vi "Keithley1a_230X_Setting.vi"(11 "YTESTER测试数据":T1) -> (3 "YTESTER结论":T2)   [LabVIEW 2017]
uses:
  YtCommon.lvlibp/yt`Step StepBaseInput.ctl
  YtCommon.lvlibp/yt`Step StepResult.ctl
  YtCommon.lvlibp/yt`Step TestData.ctl
  YtCommon.lvlibp/yt`Step System Queue.ctl
  YtCommon.lvlibp
panel:
  in  "YTESTER开放参数":T4={"YTESTER_BaseInput"={"isTest"=FALSE, "isSkip"=FALSE, "StepName"="Keithley230X设置", "OnPass"=enum."Next", "OnFail"=enum."Next", "ReTestNumber"=0.0}, "VISA resource"="", "设置选择"=enum."设置 CH1 电压&限流", "设置电压（V）"=5.0, "设置限流（mA）"=50.0}
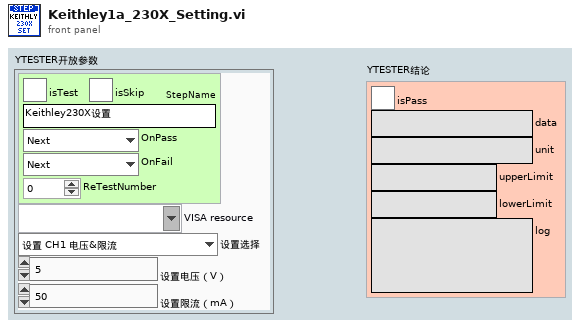
[diagram p1: front panel]
types:
  T1 = typedef "YtCommon.lvlibp/yt`Step TestData.ctl" = cluster{"Socket(From1)":i32, "SN":refnum<notifier>, "StopFlagRef":refnum<notifier>, "YT System Queue":refnum<queue>}
  T2 = typedef "YtCommon.lvlibp/yt`Step StepResult.ctl" = cluster{"isPass":bool, "data":string, "unit":string, "upperLimit":string, "lowerLimit":string, "log":string}
  T3 = typedef "YtCommon.lvlibp/yt`Step StepBaseInput.ctl" = cluster{"isTest":bool, "isSkip":bool, "StepName":string, "OnPass":enum16{"Next", "ToOVER", "Terminate"}, "OnFail":enum16{"Next", "ToOVER", "Terminate"}, "ReTestNumber":dbl}
  T4 = cluster{"YTESTER_BaseInput":T3, "VISA resource":refnum<visa-resource-name>, "设置选择":enum16{"设置 CH1 电压&限流", "设置 CH2 电压&限流", "打开 CH1", "打开 CH2", "关闭 CH1", "关闭 CH2", "打开 全部", "关闭 全部", "打开 屏显", "关闭 屏显", "查询设备（IDN？）"}, "设置电压（V）":dbl, "设置限流（mA）":dbl}
  T5 = enum16{"设置 CH1 电压&限流", "设置 CH2 电压&限流", "打开 CH1", "打开 CH2", "关闭 CH1", "关闭 CH2", "打开 全部", "关闭 全部", "打开 屏显", "关闭 屏显", "查询设备（IDN？）"}
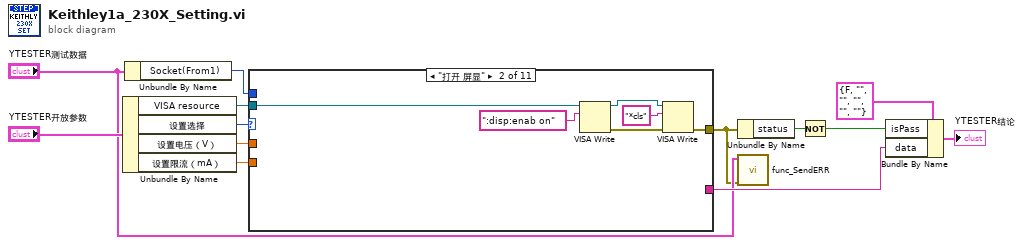
[diagram p0: block diagram]
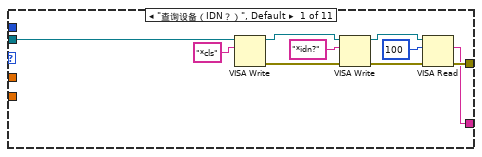
[diagram p2: hidden frame]
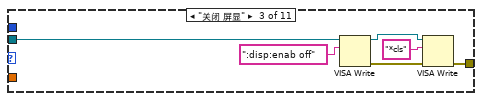
[diagram p3: hidden frame]
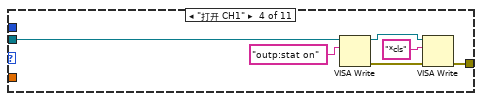
[diagram p4: hidden frame]
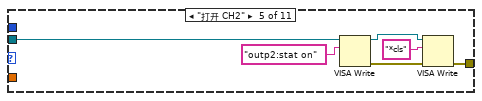
[diagram p5: hidden frame]
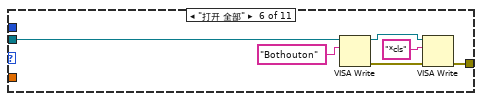
[diagram p6: hidden frame]
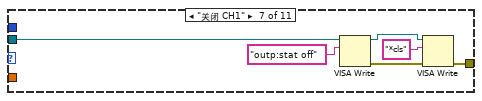
[diagram p7: hidden frame]
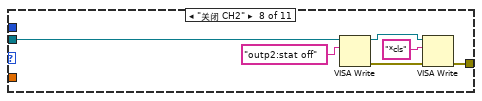
[diagram p8: hidden frame]
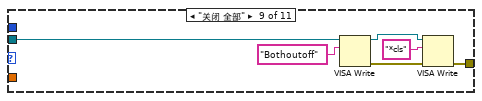
[diagram p9: hidden frame]
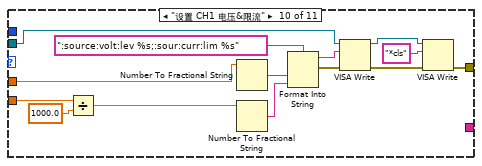
[diagram p10: hidden frame]
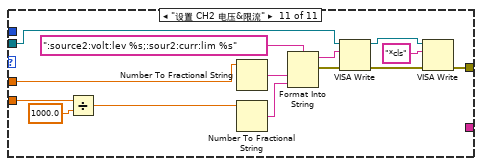
[diagram p11: hidden frame]
diagram:
  n1 = Unbundle By Name("YTESTER开放参数") -> ("VISA resource"=w9:refnum<visa-resource-name>, "设置选择"=w10:T5, "设置电压（V）"=w8:dbl, "设置限流（mA）"=w7:dbl)
  n2 = Unbundle By Name("YTESTER测试数据") -> ("Socket(From1)"=w4:i32)
  n3 = case shown="\"打开 屏显\"" w10 {
    tunnel: w9 -> [w16 w24 w31 w36 w43 w50 w55 w61 w67 w73 w89]
    tunnel: [w15 w25 w30 w37 w42 w48 w54 w60 w66 w72 w86] -> w3
    tunnel: w8 -> [_ _ _ _ _ _ _ _ _ w82 w88]
    tunnel: w7 -> [_ _ _ _ _ _ _ _ _ w79 w87]
    tunnel: [w14 _ _ _ _ _ _ _ _ _ _] -> w6
    tunnel: w4 -> [_ _ _ _ _ _ _ _ _ _ _]
    frame "查询设备（IDN？）", Default {
      n4 = VISA Write(VISA resource name=w16, write buffer="*cls") -> (VISA resource name out=w22:refnum<visa-resource-name>, error out=w18:errorcluster)  [unwired: 1 in, 1 out]
      n5 = VISA Write(VISA resource name=w22, write buffer="*idn?", error in (no error)=w18) -> (VISA resource name out=w20:refnum<visa-resource-name>, error out=w19:errorcluster)  [unwired: 1 out]
      n6 = VISA Read(VISA resource name=w20, byte count=u32 100, error in (no error)=w19) -> (read buffer=w14:string, error out=w15:errorcluster)  [unwired: 2 out]
    }
    frame "打开 屏显" {
      n7 = VISA Write(VISA resource name=w24, write buffer=":disp:enab on") -> (VISA resource name out=w28:refnum<visa-resource-name>, error out=w27:errorcluster)  [unwired: 1 in, 1 out]
      n8 = VISA Write(VISA resource name=w28, write buffer="*cls", error in (no error)=w27) -> (error out=w25:errorcluster)  [unwired: 2 out]
    }
    frame "关闭 屏显" {
      n9 = VISA Write(VISA resource name=w31, write buffer=":disp:enab off") -> (VISA resource name out=w34:refnum<visa-resource-name>, error out=w33:errorcluster)  [unwired: 1 in, 1 out]
      n10 = VISA Write(VISA resource name=w34, write buffer="*cls", error in (no error)=w33) -> (error out=w30:errorcluster)  [unwired: 2 out]
    }
    frame "打开 CH1" {
      n11 = VISA Write(VISA resource name=w36, write buffer="outp:stat on") -> (VISA resource name out=w40:refnum<visa-resource-name>, error out=w38:errorcluster)  [unwired: 1 in, 1 out]
      n12 = VISA Write(VISA resource name=w40, write buffer="*cls", error in (no error)=w38) -> (error out=w37:errorcluster)  [unwired: 2 out]
    }
    frame "打开 CH2" {
      n13 = VISA Write(VISA resource name=w43, write buffer="outp2:stat on") -> (VISA resource name out=w46:refnum<visa-resource-name>, error out=w44:errorcluster)  [unwired: 1 in, 1 out]
      n14 = VISA Write(VISA resource name=w46, write buffer="*cls", error in (no error)=w44) -> (error out=w42:errorcluster)  [unwired: 2 out]
    }
    frame "打开 全部" {
      n15 = VISA Write(VISA resource name=w50, write buffer="Bothouton") -> (VISA resource name out=w52:refnum<visa-resource-name>, error out=w51:errorcluster)  [unwired: 1 in, 1 out]
      n16 = VISA Write(VISA resource name=w52, write buffer="*cls", error in (no error)=w51) -> (error out=w48:errorcluster)  [unwired: 2 out]
    }
    frame "关闭 CH1" {
      n17 = VISA Write(VISA resource name=w55, write buffer="outp:stat off") -> (VISA resource name out=w58:refnum<visa-resource-name>, error out=w56:errorcluster)  [unwired: 1 in, 1 out]
      n18 = VISA Write(VISA resource name=w58, write buffer="*cls", error in (no error)=w56) -> (error out=w54:errorcluster)  [unwired: 2 out]
    }
    frame "关闭 CH2" {
      n19 = VISA Write(VISA resource name=w61, write buffer="outp2:stat off") -> (VISA resource name out=w64:refnum<visa-resource-name>, error out=w62:errorcluster)  [unwired: 1 in, 1 out]
      n20 = VISA Write(VISA resource name=w64, write buffer="*cls", error in (no error)=w62) -> (error out=w60:errorcluster)  [unwired: 2 out]
    }
    frame "关闭 全部" {
      n21 = VISA Write(VISA resource name=w67, write buffer="Bothoutoff") -> (VISA resource name out=w70:refnum<visa-resource-name>, error out=w69:errorcluster)  [unwired: 1 in, 1 out]
      n22 = VISA Write(VISA resource name=w70, write buffer="*cls", error in (no error)=w69) -> (error out=w66:errorcluster)  [unwired: 2 out]
    }
    frame "设置 CH1 电压&限流" {
      n23 = Divide(x=w79, y=1000.0 ("x")) -> (x/y=w81:dbl)
      n24 = Number To Fractional String(number=w82) -> (F-format string=w77:string)  [unwired: 3 in]
      n25 = Number To Fractional String(number=w81) -> (F-format string=w76:string)  [unwired: 3 in]
      n26 = Format Into String(format string=":source:volt:lev %s;:sour:curr:lim %s" ("write buffer"), w77, w76) -> (resulting string=w75:string, error out=w74:errorcluster)  [unwired: 2 in]
      n27 = VISA Write(VISA resource name=w73, write buffer=w75, error in (no error)=w74) -> (VISA resource name out=w84:refnum<visa-resource-name>, error out=w83:errorcluster)  [unwired: 1 out]
      n28 = VISA Write(VISA resource name=w84, write buffer="*cls", error in (no error)=w83) -> (error out=w72:errorcluster)  [unwired: 2 out]
    }
    frame "设置 CH2 电压&限流" {
      n29 = Divide(x=w87, y=1000.0 ("x")) -> (x/y=w96:dbl)
      n30 = Number To Fractional String(number=w88) -> (F-format string=w93:string)  [unwired: 3 in]
      n31 = Number To Fractional String(number=w96) -> (F-format string=w92:string)  [unwired: 3 in]
      n32 = Format Into String(format string=":source2:volt:lev %s;:sour2:curr:lim %s" ("write buffer"), w93, w92) -> (resulting string=w91:string, error out=w90:errorcluster)  [unwired: 2 in]
      n33 = VISA Write(VISA resource name=w89, write buffer=w91, error in (no error)=w90) -> (VISA resource name out=w98:refnum<visa-resource-name>, error out=w97:errorcluster)  [unwired: 1 out]
      n34 = VISA Write(VISA resource name=w98, write buffer="*cls", error in (no error)=w97) -> (error out=w86:errorcluster)  [unwired: 2 out]
    }
  }
  n35 = Unbundle By Name(w3) -> ("status"=w2:bool)
  n36 = call "func_SendERR.vi"("ERR (String\\Errclust)"=w3, "YTESTER测试数据 in"="YTESTER测试数据") -> ()  [unwired: 9 in, 1 out]
  n37 = Not(x=w2) -> (.not. x?=w1:bool)
  n38 = Bundle By Name(cluster=T2 {"isPass"=FALSE, "data"="", "unit"="", "upperLimit"="", "lowerLimit"="", "log"=""} ("Result"), "isPass"=w1, "data"=w6) -> (→"YTESTER结论":T2)
